vi "Datasheet Generate Table Data.vi"(8 "error in (no error)":errorcluster, 10 "Data Tree":T1[][](array[typedef]), 11 "Column Data":T9[](array[typedef])) -> (0 "error out":errorcluster, 1 "First item":string, 2 "Comma rows":string, 3 "HTM Table Row":string)   [LabVIEW 2011]
uses:
  Column Data.ctl
  TDMS/TDMS Model Number.ctl
  TDMS/TDMS Serial Number.ctl
  TDMS/TDMS File.ctl
  TDMS/TDMS Run.ctl
  TDMS/TDMS Channel (Sxx).ctl
  database/Fields/Field Record.ctl
  database/Fields/Field DataTypes.ctl
  database/Fields/Field NextItem.ctl
panel:
  out "time":u32
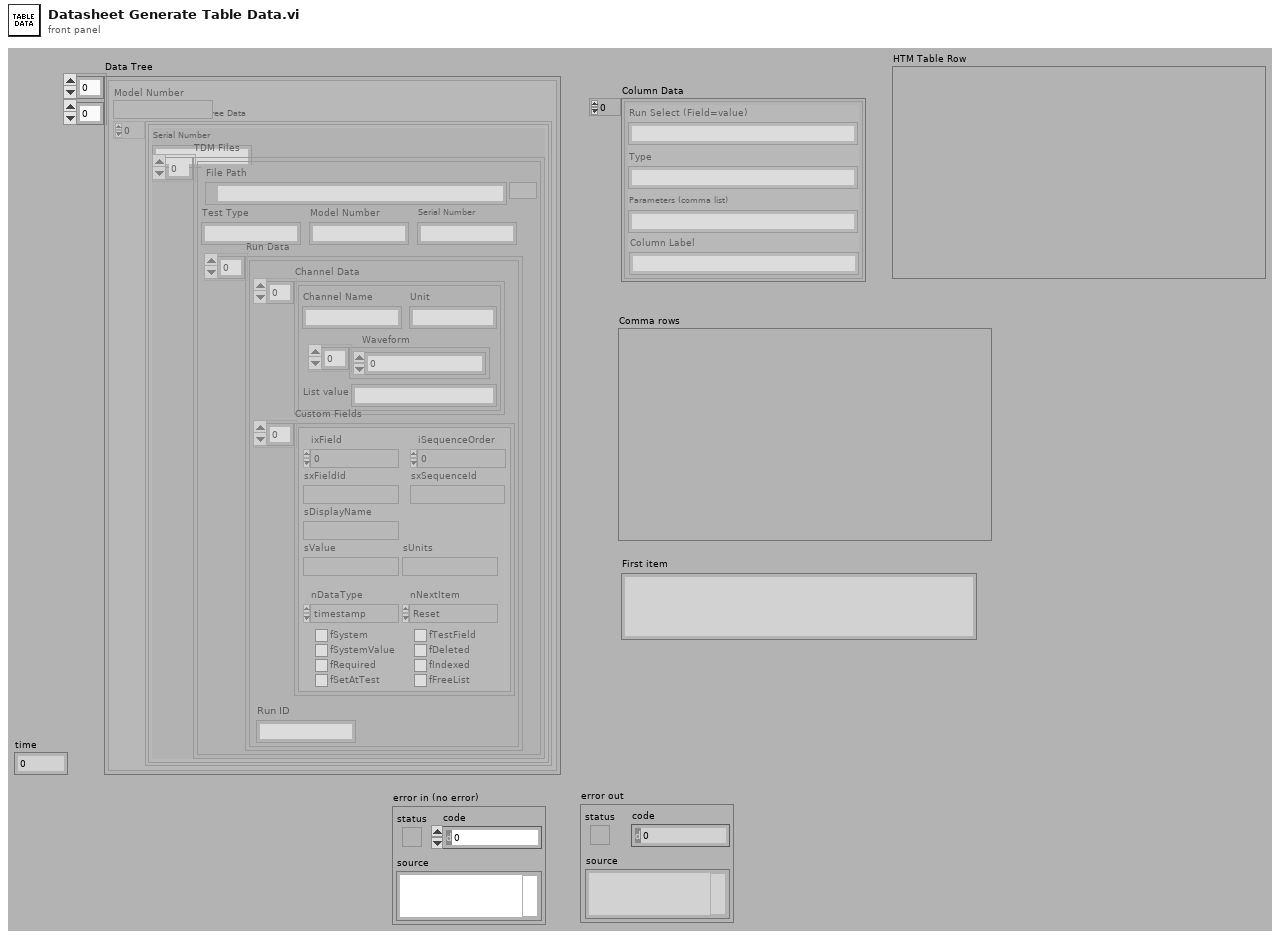
[diagram p1: front panel]
types:
  T1 = typedef "TDMS Model Number.ctl" = cluster{"Model Number":string, "Serial Number Tree Data":T2[]}
  T2 = typedef "TDMS Serial Number.ctl" = cluster{"Serial Number":string, "TDM Files":T3[]}
  T3 = typedef "TDMS File.ctl" = cluster{"File Path":path, "Run Data":T4[], "Serial Number":string, "Model Number":string, "Test Type":string}
  T4 = typedef "TDMS Run.ctl" = cluster{"Channel Data":T5[], "Custom Fields":T6[], "Run ID":string}
  T5 = typedef "TDMS Channel (Sxx).ctl" = cluster{"Channel Name":string, "Waveform":dbl[], "Unit":string, "List value":string}
  T6 = typedef "Field Record.ctl" = cluster{"ixField":i32, "iSequenceOrder":i32, "sxFieldId":string, "sxSequenceId":string, "sDisplayName":string, "sValue":string, "sUnits":string, "nDataType":T7, "nNextItem":T8, "fSystem":bool, "fSystemValue":bool, "fRequired":bool, "fSetAtTest":bool, "fTestField":bool, "fDeleted":bool, "fIndexed":bool, "fFreeList":bool}
  T7 = typedef "Field DataTypes.ctl" = enum32{"text", "numeric", "list", "timestamp", "boolean"}
  T8 = typedef "Field NextItem.ctl" = enum32{"Reset", "Retain", "Auto-Increment"}
  T9 = typedef "Column Data.ctl" = cluster{"Run Select (Field=value)":string, "Type":string, "Parameters (comma list)":string, "Column Label":string}
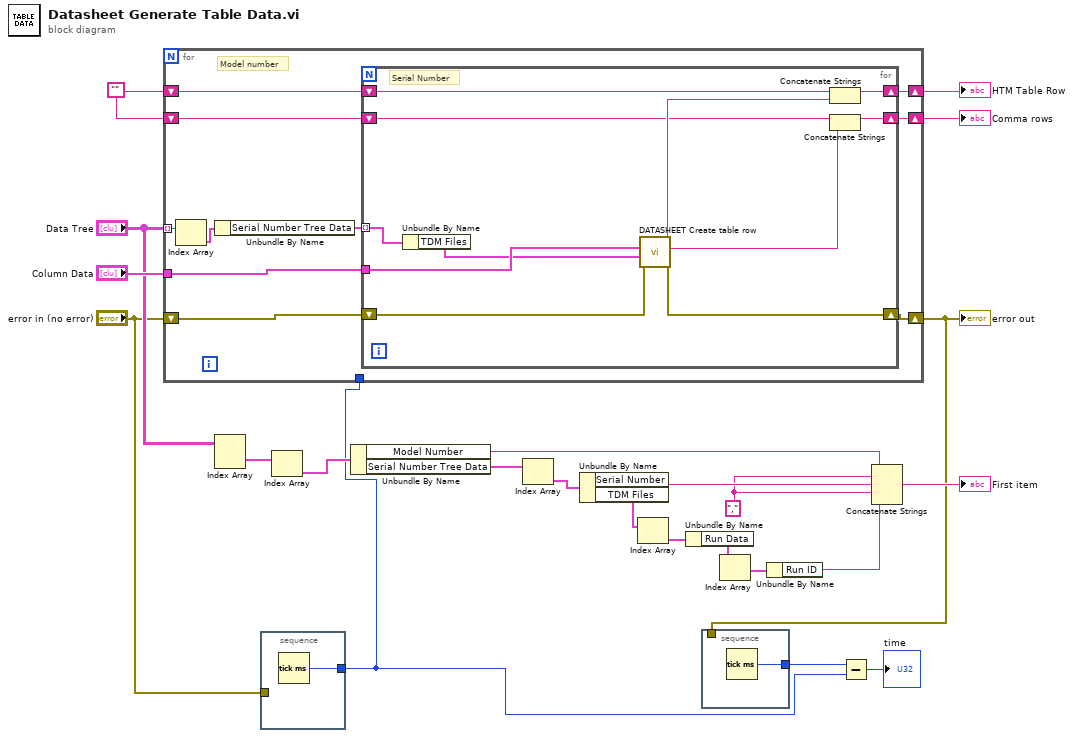
[diagram p0: block diagram]
diagram:
  w9 = ","
  w21 = ""
  n1 = Index Array(array="Data Tree") -> (element=w18:T1[])  [unwired: 2 in]
  n2 = stacked-sequence {
    tunnel: [w24] -> w2
    tunnel: "error in (no error)" -> [_]
    frame #0 {
      n3 = Tick Count (ms)() -> (millisecond timer value=w24:u32)
    }
  }
  n4 = for {
    tunnel: "Column Data" -> [w34]
    tunnel: "Data Tree" -> [w31] mode=indexing
    shift-right: [w33] -> w22
    shift-left: w21 -> [w32]
    shift-right: [w29] -> w4
    shift-left: "error in (no error)" -> [w28]
    shift-right: [w26] -> w20
    shift-left: w21 -> [w27]
    tunnel: w2 -> [_]
    # "Model number"
    n5 = Index Array(array=w31) -> (element=w25:T1)  [unwired: 1 in]
    n6 = Unbundle By Name(w25) -> ("Serial Number Tree Data"=w30:T2[])
    n7 = for {
      tunnel: w34 -> [w42]
      shift-right: [w44] -> w33
      shift-left: w32 -> [w45]
      tunnel: w30 -> [w43] mode=indexing
      shift-right: [w39] -> w29
      shift-left: w28 -> [w38]
      shift-right: [w37] -> w26
      shift-left: w27 -> [w36]
      # "Serial Number"
      n8 = Unbundle By Name(w43) -> ("TDM Files"=w41:T3[])
      n9 = call "DATASHEET Create table row.vi"("error in (no error)"=w38, "TDM Data"=w41, "Columns"=w42) -> ("error out"=w39:errorcluster, "Comma row"=w35:string, "HTM Row"=w40:string)  [unwired: 3 in, 3 out]
      n10 = Concatenate Strings(w45, w40) -> (w44:string)
      n11 = Concatenate Strings(w36, w35) -> (w37:string)
    }
  }
  "HTM Table Row" <- w22
  "error out" <- w4
  "Comma rows" <- w20
  n12 = Index Array(array=w18) -> (element=w3:T1)  [unwired: 1 in]
  n13 = Unbundle By Name(w3) -> ("Model Number"=w15:string, "Serial Number Tree Data"=w17:T2[])
  n14 = Index Array(array=w17) -> (element=w16:T2)  [unwired: 1 in]
  n15 = Unbundle By Name(w16) -> ("Serial Number"=w14:string, "TDM Files"=w12:T3[])
  n16 = Index Array(array=w12) -> (element=w11:T3)  [unwired: 1 in]
  n17 = Unbundle By Name(w11) -> ("Run Data"=w10:T4[])
  n18 = stacked-sequence {
    tunnel: [w46] -> w6
    tunnel: w4 -> [_]
    frame #0 {
      n19 = Tick Count (ms)() -> (millisecond timer value=w46:u32)
    }
  }
  n20 = Index Array(array=w10) -> (element=w8:T4)  [unwired: 1 in]
  n21 = Unbundle By Name(w8) -> ("Run ID"=w7:string)
  n22 = Subtract(x=w6, y=w2) -> (x-y=→"time":u32)
  n23 = Concatenate Strings(w15, w9, w14, w9, w7) -> (→"First item":string)
